vi "GPIB_autodetect.vi"(7 "ID command":string, 8 "error in (no error)":errorcluster, 10 "Instrument address in":refnum<visa-resource-name>, 11 "InstrControl in":refnum<class "InstrControl.lvclass">) -> (0 "error out":errorcluster, 2 "Instrument address out":refnum<visa-resource-name>, 3 "InstrControl out":refnum<class "InstrControl.lvclass">)   [LabVIEW 2013, in "InstrControl.lvclass"]
uses:
  InstrControl.lvclass
panel:
  out "addresses found":string[](array[string])
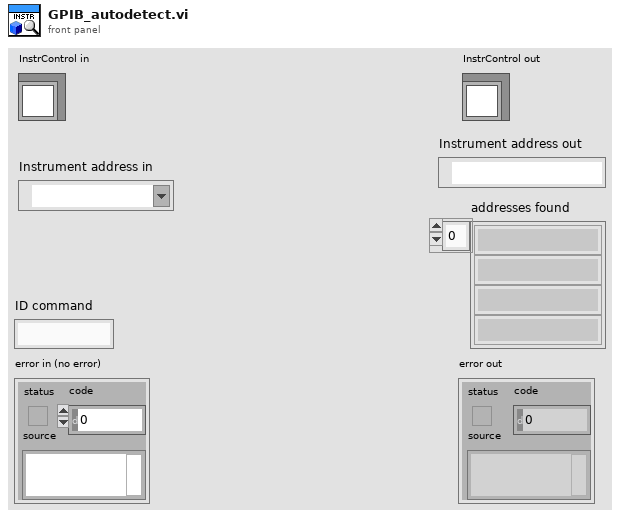
[diagram p1: front panel]
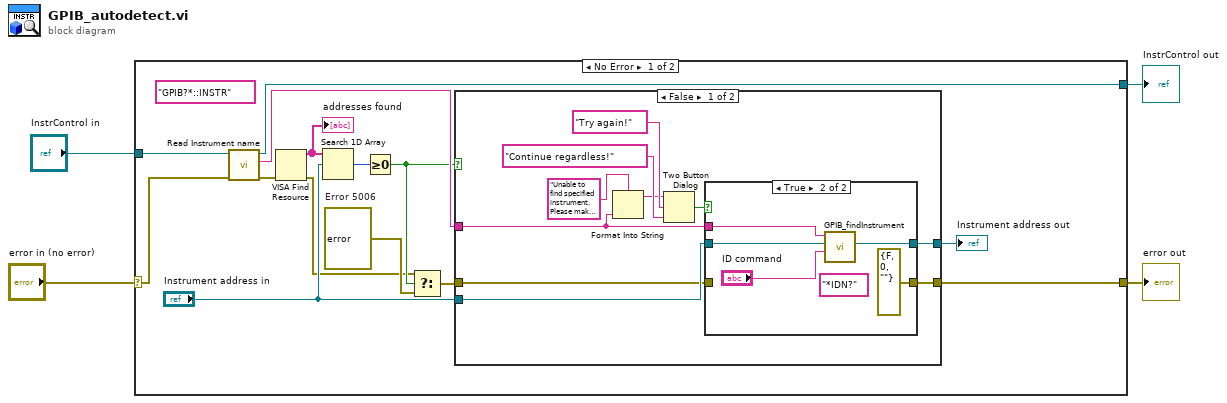
[diagram p0: block diagram]
diagram:
  n1 = case shown="No Error" "error in (no error)" {
    selector: "error in (no error)" -> [w17 w39]
    tunnel: [w14 w39] -> w3
    tunnel: [w16 w38] -> w1
    tunnel: "InstrControl in" -> [w18 w38]
    frame No Error {
      w12 = errorcluster {"status"=FALSE, "code"=5005, "source"="Unable to find specified instrument.  Please make sure the it is connected to your system and switched on."}  # Error 5006
      (unwired) "GPIB?*::INSTR" ("expression (\"\")")
      n2 = call-dynamic "Read Instrument name.vi"("error in (no error)"=w17, "InstControl in"=w18) -> ("error out"=w15:errorcluster, "Instrument name"=w13:string, "InstControl out"=w16:refnum<class "InstrControl.lvclass">)  [unwired: 7 in]
      n3 = VISA Find Resource(8:w15) -> (0:w5:errorcluster, 3:w6:string[])  [unwired: 2 in, 1 out]
      "addresses found" <- w6
      n4 = Search 1D Array(1D array=w6, element="Instrument address in") -> (index of element=w10:i32)  [unwired: 1 in]
      n5 = Greater Or Equal To 0?(x=w10) -> (x >= 0?=w9:bool)
      n6 = Select(t=w5, s=w9, f=w12) -> (s? t:f=w7:errorcluster)
      n7 = case shown="False" w9 {
        tunnel: "Instrument address in" -> [w25 w37]
        tunnel: [w24 w37] -> w11
        tunnel: w7 -> [w23 w36]
        tunnel: [w22 w36] -> w14
        tunnel: w13 -> [w20 _]
        frame False {
          n8 = Format Into String(format string="Unable to find specified instrument.  Please make sure the it is connected to your system and switched on.\n\n%s" ("source"), w20) -> (resulting string=w19:string)  [unwired: 2 in, 1 out]
          n9 = Two Button Dialog(message=w19, 1:"Continue regardless!", 2:"Try again!") -> (T button?=w26:bool)
          n10 = case shown="True" w26 {
            tunnel: w25 -> [w30 w35]
            tunnel: [w30 w34] -> w24
            tunnel: w23 -> [w29 _]
            tunnel: [w29 errorcluster {"status"=FALSE, "code"=0, "source"=""} ("error constant")] -> w22
            tunnel: w20 -> [_ w32]
            frame False {
            }
            frame True {
              (unwired) "*IDN?" ("regular expression")
              n11 = call "GPIB_findInstrument.vi"("ID command"="ID command", "revised Instrument address"=w35, "Instrument name IN"=w32) -> ("revised GPIB address OUT"=w34:refnum<visa-resource-name>)  [unwired: 8 in]
            }
          }
        }
        frame True {
        }
      }
      "Instrument address out" <- w11
    }
    frame Error {
    }
  }
  "error out" <- w3
  "InstrControl out" <- w1
